vi "Find A Zero.vi"(9 "Ccovered":bool[](array[boolean]), 10 "Rcovered":bool[](array[boolean]), 11 "Matrix":T1) -> (1 "Column":i32, 2 "Row":i32, 3 "Matrix Out":T1)   [LabVIEW 2013]
uses:
  <vilib>/Analysis/Matrix/Datatypes/RealMatrix.ctl
  <vilib>/Analysis/Matrix/NI_Matrix.lvlib
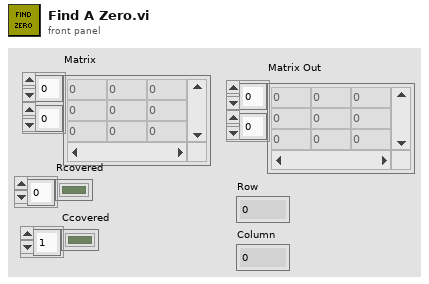
[diagram p1: front panel]
types:
  T1 = typedef "NI_Matrix.lvlib/RealMatrix.ctl" = dbl[][]
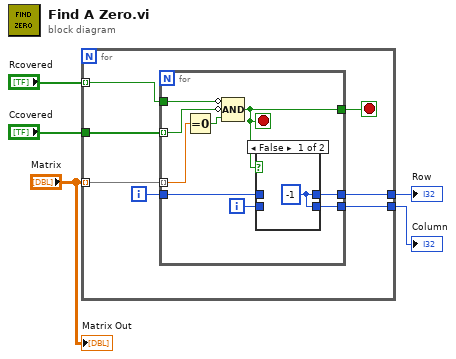
[diagram p0: block diagram]
diagram:
  n1 = for {
    tunnel: "Matrix" -> [w10] mode=indexing
    tunnel: "Rcovered" -> [w12] mode=indexing
    tunnel: "Ccovered" -> [w11]
    tunnel: [w7] -> w2
    tunnel: [w6] -> w1
    i -> [w8]
    stop <- w9 stop-if-true
    n2 = for {
      tunnel: w12 -> [w18]
      tunnel: w11 -> [w19] mode=indexing
      tunnel: w10 -> [w21] mode=indexing
      tunnel: [w17] -> w9
      tunnel: w8 -> [w16]
      tunnel: [w14] -> w7
      tunnel: [w13] -> w6
      i -> [w15]
      stop <- w17 stop-if-true
      n3 = Equal To 0?(x=w21) -> (x = 0?=w20:bool)
      n4 = Compound Arithmetic op=AND(invert w18, invert w19, w20) -> (w17:bool)
      n5 = case shown="False" w17 {
        tunnel: w16 -> [_ w24]
        tunnel: w15 -> [_ w23]
        tunnel: [w22 w24] -> w14
        tunnel: [w22 w23] -> w13
        frame False {
          w22 = -1
        }
        frame True {
        }
      }
    }
  }
  "Row" <- w2
  "Column" <- w1
  "Matrix Out" <- "Matrix"
